vi "_OLS_Main_Rev3.vi"() -> ()   [LabVIEW 2024]
uses:
  Control Definitions/Def Results2.ctl
  Control Definitions/Def_ATPStatus.ctl
  Control Definitions/Def_PumpSpeed.ctl
  Control Definitions/Def TestState.ctl
  Control Definitions/DEF_CalConstants.ctl
  Control Definitions/Def PumpCtlRefs.ctl
  Control Definitions/Def CalTable.ctl
  Control Definitions/Def CalCoef.ctl
  Control Definitions/Registry Keys.ctl
  Control Definitions/Global 2.vi
  Control Definitions/Global 1.vi
panel:
  out "Cal Coef":T1
  in  "Cal Table":T2={"Level"={"LSf"=0.0, "LMf"=0.0, "LKf"=0.0, "LMe"=0.0, "LKe"=0.0, "LSe"=0.0}, "DataQ CH"=[{"RqLA"=0.5698, "RmLA"=102.56, "RqHA"=5.58, "RmHA"=981.0}, {"RqLA"=0.5707, "RmLA"=102.56, "RqHA"=5.5902, "RmHA"=978.2}]}
  out "ItemPath":string
  out "Laser (raw) 2":dbl=2.1254169074046554
  in  "End Prog":bool
  out "Test Index Out":i32=4
  out "PumpCtlRef out":T3
  out "Reg Cal Constants":T4={"Measure High"="0.000", "Laser High"="5.419", "Measure Low"="0.000", "Laser Low"="5.419", "Cal Name"="Rick", "Cal Date"="8/13/2024 3:15:10 PM", "Empty Inches"=8.0, "Full Inches"=2.6, "Valid"=FALSE}
  in  "Skip Pre-Lube":bool=TRUE
  out "TEST State Out":T5=enum."Wait1"
  in  "Pump Speed":T6=enum."STOP"
  in  "Num Chan":i32=2
  in  "VISA Refnum in":refnum<visa-resource-name>="COM3"
  in  "SimPV":bool
  out "Ch B  Sim":dbl=101.0
  out "Ch A  Sim":dbl=200.0
  out "Root Path":path=path "M:/OLS Level Test Project/PWC-OLS-Rev2/PWC-OLS"
  out "Time(ms)":dbl=7.099999999999983
  out "Level":bool=TRUE
  out "DataQ":bool
  in  "ChA":dbl(slide)=24.489795918367346 scale=0.0..1200.0
  in  "ChB":dbl(slide)=36.73469387755102 scale=0.0..1200.0
  in  "ChB +100":bool
  in  "ChA +100":bool
  in  "Check":bool
  out "Laser (raw)":dbl=2.1254169074046554
  out "Results out":T7=[[{"Fill"=0.0, "Drain"=0.0, "Status"=0, "Resistor"=100.0}, {"Fill"=8.52, "Drain"=0.0, "Status"=0, "Resistor"=101.0}], [{"Fill"=7.50499999999993, "Drain"=0.0, "Status"=4, "Resistor"=200.0}, {"Fill"=7.27499999999994, "Drain"=0.0, "Status"=0, "Resistor"=0.0}], [{"Fill"=0.0, "Drain"=0.0, "Status"=0, "Resistor"=0.0}, {"Fill"=0.0, "Drain"=0.0, "Status"=0, "Resistor"=0.0}], [{"Fill"=0.0, "Drain"=0.0, "Status"=0, "Resistor"=0.0}, {"Fill"=0.0, "Drain"=0.0, "Status"=0, "Resistor"=0.0}], [{"Fill"=0.0, "Drain"=0.0, "Status"=0, "Resistor"=0.0}, {"Fill"=0.0, "Drain"=0.0, "Status"=0, "Resistor"=0.0}], [{"Fill"=0.0, "Drain"=0.0, "Status"=0, "Resistor"=0.0}, {"Fill"=0.0, "Drain"=0.0, "Status"=0, "Resistor"=0.0}], [{"Fill"=0.0, "Drain"=0.0, "Status"=0, "Resistor"=0.0}, {"Fill"=0.0, "Drain"=0.0, "Status"=0, "Resistor"=0.0}], [{"Fill"=0.0, "Drain"=0.0, "Status"=0, "Resistor"=0.0}, {"Fill"=0.0, "Drain"=0.0, "Status"=0, "Resistor"=0.0}], [{"Fill"=0.0, "Drain"=0.0, "Status"=0, "Resistor"=0.0}, {"Fill"=0.0, "Drain"=0.0, "Status"=0, "Resistor"=0.0}], [{"Fill"=0.0, "Drain"=0.0, "Status"=0, "Resistor"=0.0}, {"Fill"=0.0, "Drain"=0.0, "Status"=0, "Resistor"=0.0}], [{"Fill"=0.0, "Drain"=0.0, "Status"=0, "Resistor"=0.0}, {"Fill"=0.0, "Drain"=0.0, "Status"=0, "Resistor"=0.0}]] {"Resistor" format="%.1f"; "Drain" format="%.3f"; "Fill" format="%.3f"}
  in  "DUT":i16=1
  in  "Pump JOG":bool
  in  "Run Test":bool=TRUE
  in  "Normal":cluster{u32, u32}[](array[cluster])=[{16711680, 1244948}]
  in  "Sim Color":cluster{u32, u32}[](array[cluster])=[{16774656, 1244948}]
  out "Level \nStatus":bool=TRUE
  out "DataQ\nStatus":bool
  in  "Level SP":dbl(slide)=7.46 scale=8.5..2.0
  in  "Level PV":dbl(slide)=7.459999999999936 scale=8.5..2.0
  out "Level":dbl=7.459999999999936 format="%.3f"
  in  "Drain":bool
  in  "Fill":bool
  in  "Simulate":bool=TRUE
  out "TEST NME":string="OLR001--"
  out "DataQ Input":T9(graph)={"ChA Ohms"=200.0, "ChB Ohms"=101.0, "Laser (raw)"=2.1254169074046554}
  out "Time Stamp":timestamp=timestamp(3807627813.1312256 s since 1904-01-01)
  in  "stop":bool
  out "ChB Ohms":dbl=101.0 format="%.1f"
  out "ChA Ohms":dbl=200.0 format="%.1f"
  # "Calibration & Scaling Table\n               Tank         Key          Ref\n               Scale        Level        Measure\nEmpty\n\n\nFull"
  # "8.5      1.7752      7.844\n\n2.0      6.112        3.511"
  # "CHA"
  # "CHB"
  # "ATP       Resistance     Fill        Drain"
  # "ATP       Resistance     Fill        Drain"
  # "Simulated Instrument Inputs"
  # "PUMP"
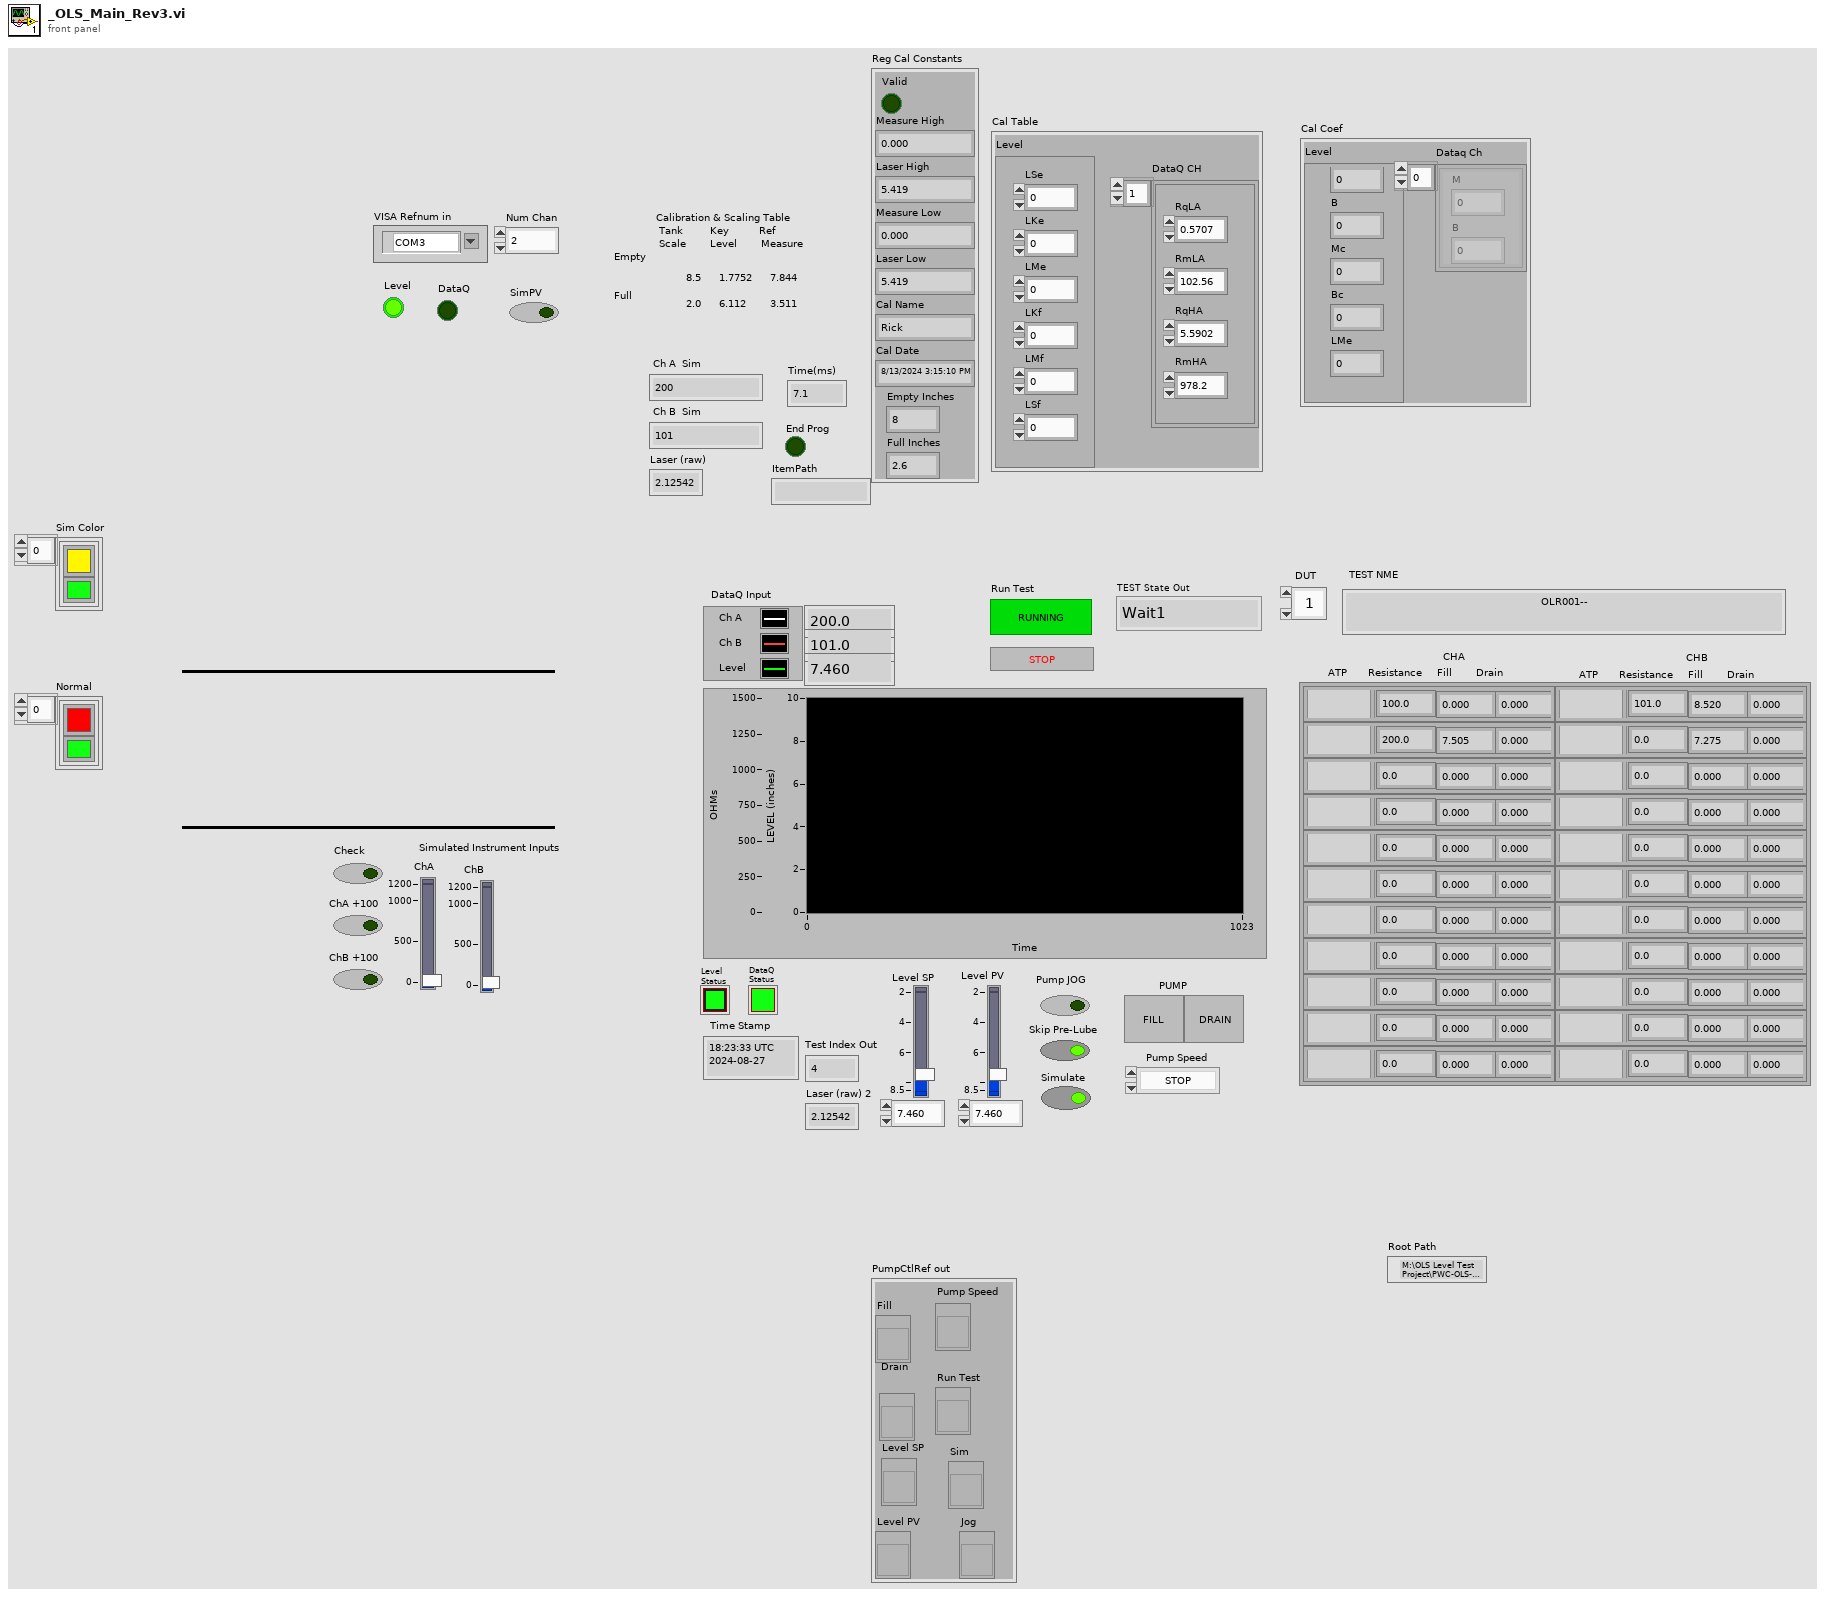
[diagram p1: front panel]
types:
  T1 = typedef "Def CalCoef.ctl" = cluster{"Level":cluster{"LMe":dbl, "Bc":dbl, "Mc":dbl, "B":dbl, "M":dbl}, "Dataq Ch":cluster{"B":dbl, "M":dbl}[]}
  T2 = typedef "Def CalTable.ctl" = cluster{"Level":cluster{"LSf":dbl, "LMf":dbl, "LKf":dbl, "LMe":dbl, "LKe":dbl, "LSe":dbl}, "DataQ CH":cluster{"RqLA":dbl, "RmLA":dbl, "RqHA":dbl, "RmHA":dbl}[]}
  T3 = typedef "Def PumpCtlRefs.ctl" = cluster{"Fill ":refnum<vi>, "Drain":refnum<vi>, "Level PV":refnum<vi>, "Pump Speed":refnum<vi>, "Run Test":refnum<vi>, "Sim":refnum<vi>, "Jog":refnum<vi>, "Level SP":refnum<vi>}
  T4 = typedef "DEF_CalConstants.ctl" = cluster{"Measure High":string, "Laser High":string, "Measure Low":string, "Laser Low":string, "Cal Name":string, "Cal Date":string, "Empty Inches":dbl, "Full Inches":dbl, "Valid":bool}
  T5 = typedef "Def TestState.ctl" = enum16{"MANUAL", "Start", "Pre-Fill", "Pre-Fill Measure", "Pre-Drain", "Pre-Drin Measure", "Init-Record", "Load Fill Spec", "Filling Hi", "Wait1", "Record Fill", "Load Drain Spec", "Draining Lo", "Wait2", "Record Drain", "Empty", "Done"}
  T6 = typedef "Def_PumpSpeed.ctl" = enum16{"FAST", "SLOW", "CREEP", "STOP"}
  T7 = typedef "Def Results2.ctl" = cluster{"Fill":dbl, "Drain":dbl, "Status":T8, "Resistor":dbl}[][]
  T8 = typedef "Def_ATPStatus.ctl" = i16
  T9 = cluster{"ChA Ohms":dbl, "ChB Ohms":dbl, "Laser (raw)":dbl}
  T10 = typedef "Registry Keys.ctl" = enum16{"Report Files Key", "Config Files Key"}
  T11 = cluster{"Level \nStatus":refnum<vi>, "DataQ\nStatus":refnum<vi>}
  T12 = typedef "Def FullCfg.ctl" = cluster{"Bench Config":T13, "Test Value Table ":dbl[][], "Table Col Titles":string[][], "cluster":T3, "Bench Status":T14}
  T13 = typedef "Def BenchCfg.ctl" = cluster{"Name":string, cluster{"Step Levels":dbl, "Tolerance":dbl, "Sample Rate":dbl, "Resistor":dbl, "M Level Cal":dbl, "[B Level Cal":dbl, "Max Fill Rate":dbl, "Empty Inches":dbl, "Full Inches":dbl}}
  T14 = typedef "Def Bench Status.ctl" = cluster{"Pump Status":refnum<vi>, "Instrumnet\n Status":refnum<vi>}
  T15 = enum16{"MANUAL", "Start", "Filling", "FULL", "Draining", "EMPTY", "Done"}
  T16 = cluster{"Resistor":dbl, "Fill":dbl, "Drain":dbl, "Status":i16}
  T17 = cluster{"Resistor":dbl, "Fill":dbl, "Drain":dbl, "Status":i16}[][]
  T18 = typedef "DEF_SpecsOut.ctl" = cluster{"aSpecsTable":T19[], "Pump CtlRef In":T3, "TEST State Out":T5, "TEST Index":i32, "Drain!Fill":bool}
  T19 = typedef "Def Spec RNG.ctl" = cluster{"Specs":dbl[], "LUT Status":T20}
  T20 = typedef "Ded LUT_Status.ctl" = cluster{"ChA/!ChB":bool, "Drain/!Fill":bool, "In Range?":bool, "Switch Range?":bool, "Measure R?":bool, "Vaild R?":bool, "Index(n)":i32, "Index(n)-1":i32, "Index Max":i32, "Index(n-1)":i32}
  T21 = typedef "Def Measure.ctl" = cluster{"ChA R":dbl, "ChB R":dbl, "Level PV":dbl}
  T22 = cluster{"Resistor":dbl, "Fill":dbl, "Drain":dbl, "Resistor":dbl}[][]
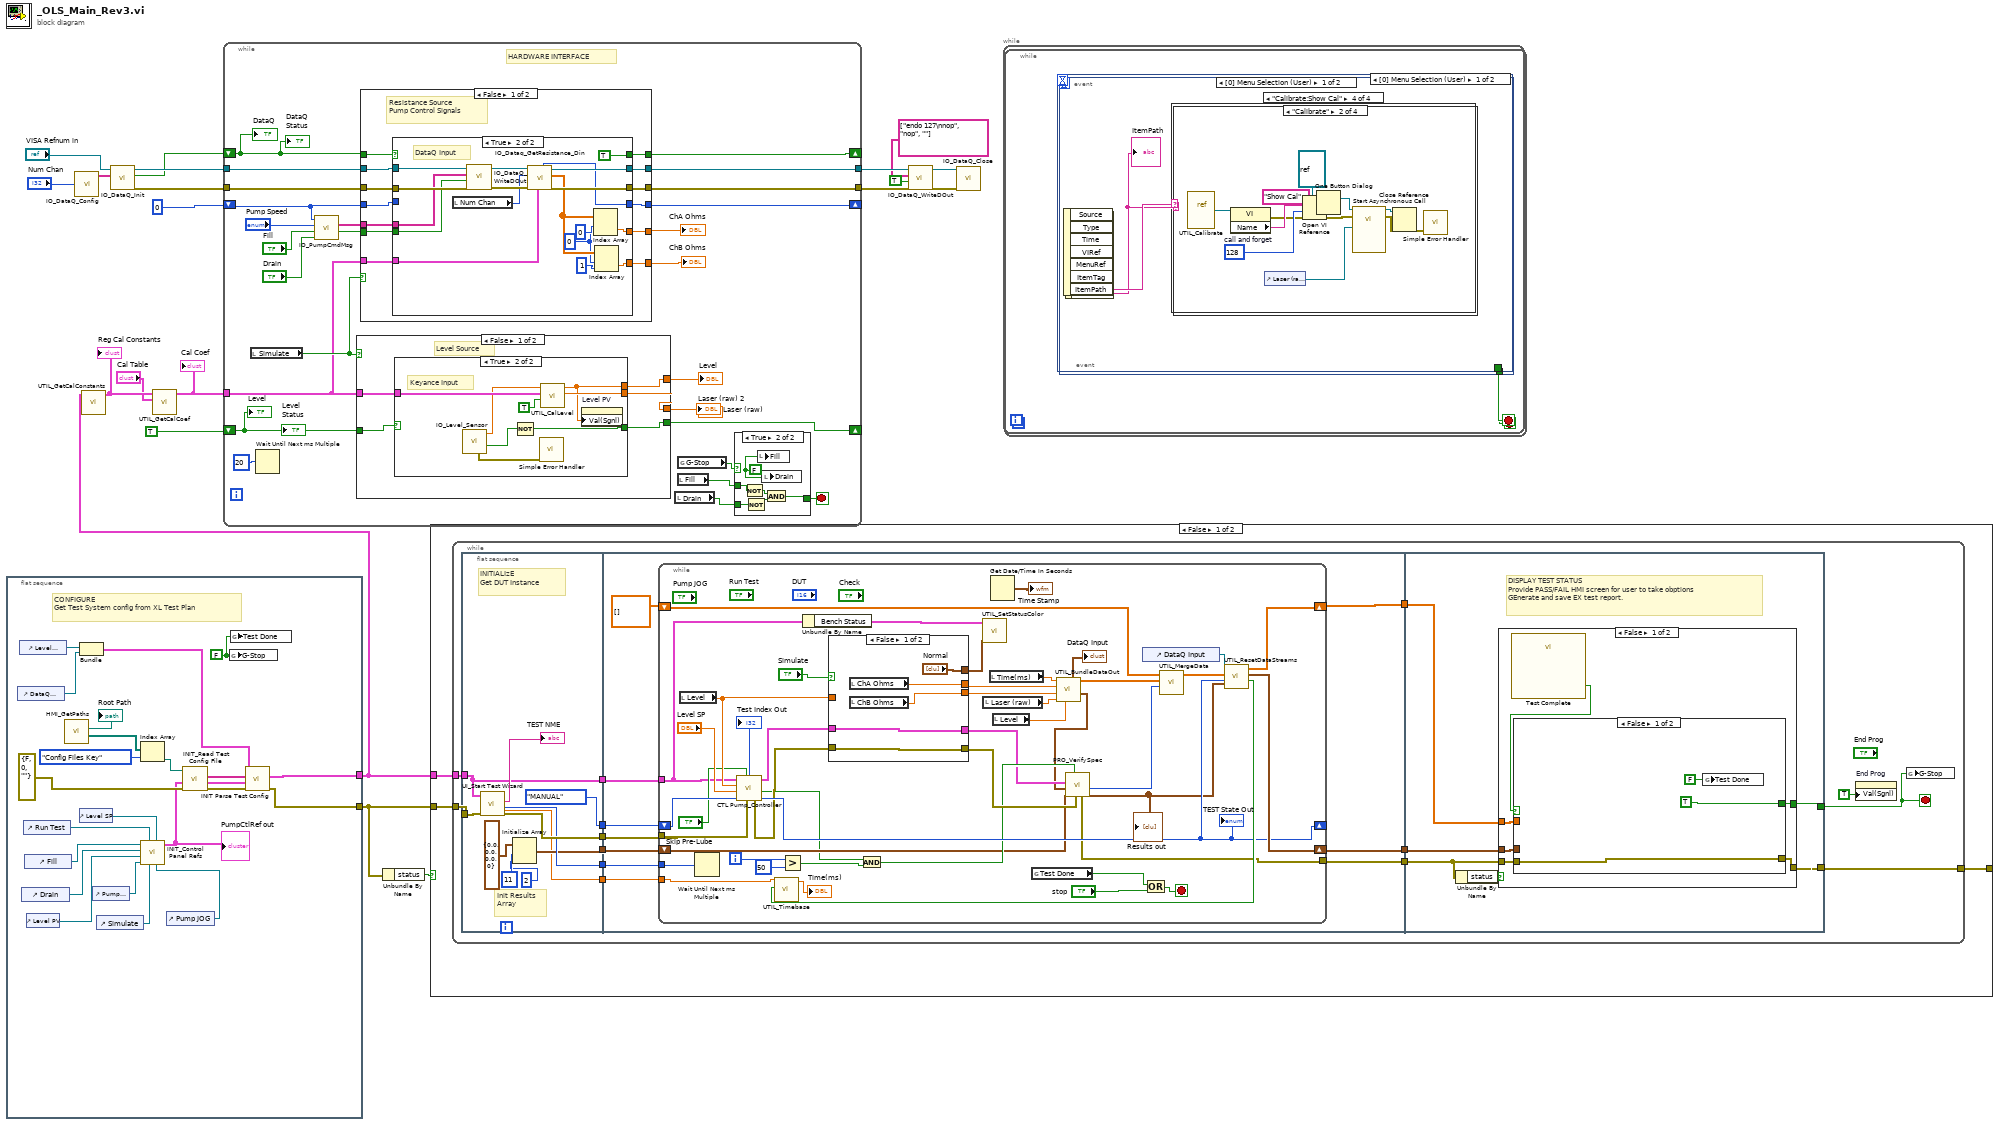
[diagram p0: block diagram]
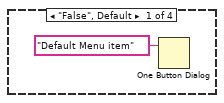
[diagram p2: hidden frame]
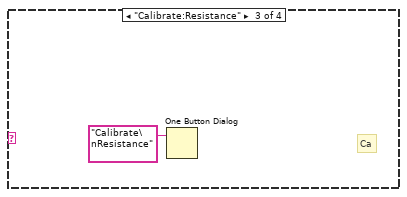
[diagram p3: hidden frame]
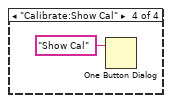
[diagram p4: hidden frame]
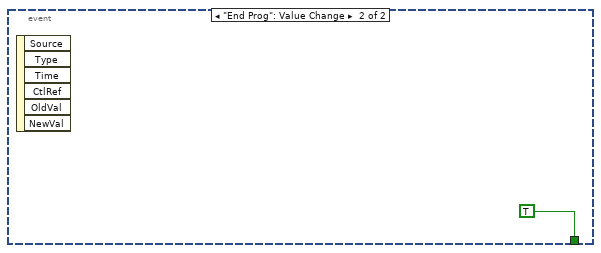
[diagram p5: hidden frame]
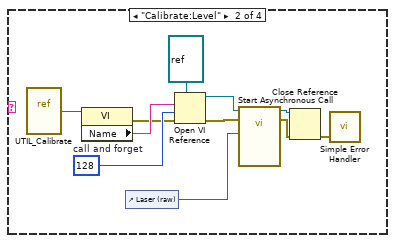
[diagram p7: hidden frame]
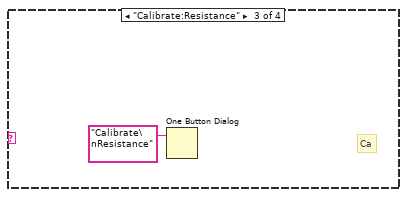
[diagram p8: hidden frame]
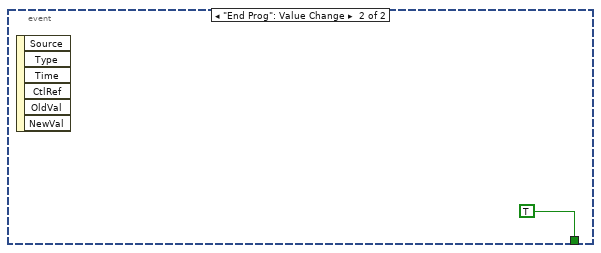
[diagram p9: hidden frame]
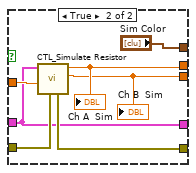
[diagram p10: hidden frame]
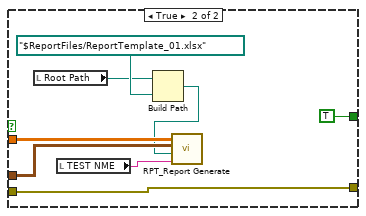
[diagram p11: hidden frame]
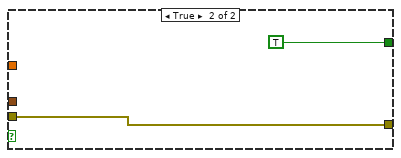
[diagram p12: hidden frame]
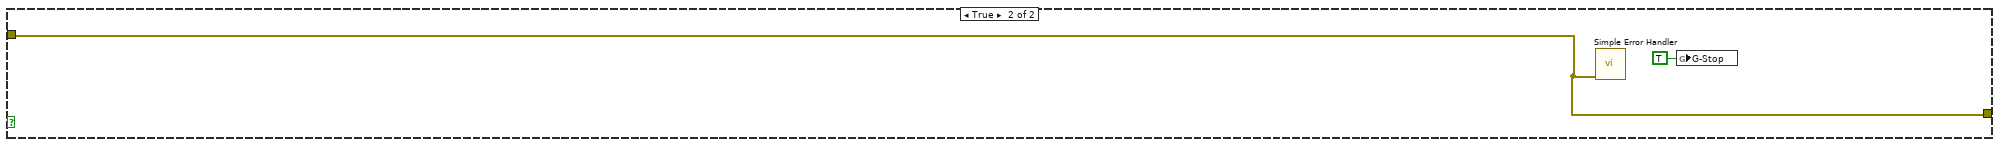
[diagram p13: hidden frame]
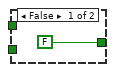
[diagram p14: hidden frame]
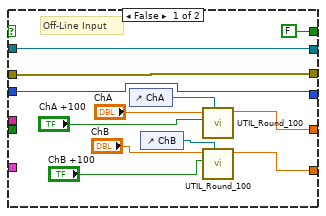
[diagram p15: hidden frame]
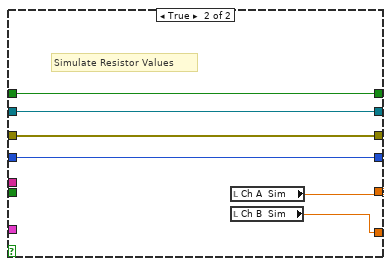
[diagram p16: hidden frame]
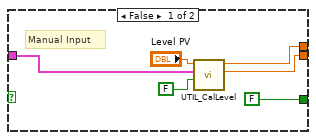
[diagram p17: hidden frame]
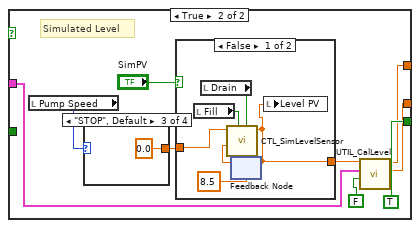
[diagram p18: hidden frame]
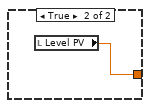
[diagram p19: hidden frame]
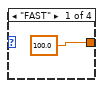
[diagram p20: hidden frame]
diagram:
  n1 = flat-sequence {
    tunnel: [w40] -> w14
    tunnel: [w32] -> w3
    frame #0 {
      w27 = FALSE ("G-Stop")
      # "CONFIGURE\nGet Test System config from XL Test Plan"
      n2 = control-ref of="DataQ\nStatus"() -> (w29:refnum<vi>)
      n3 = control-ref of="Level \nStatus"() -> (w39:refnum<vi>)
      n4 = control-ref of="Drain"() -> (w41:refnum<vi>)
      n5 = control-ref of="Run Test"() -> (w34:refnum<vi>)
      n6 = control-ref of="Fill"() -> (w35:refnum<vi>)
      n7 = control-ref of="Level PV"() -> (w37:refnum<vi>)
      n8 = call "HMI_GetPaths.vi"() -> ("Default Paths"=w22:path[], "Root Path"=→"Root Path":path)  [unwired: 10 in]
      n9 = Bundle("Level \nStatus"=w39, "DataQ\nStatus"=w29) -> (w38:T11)  [unwired: 1 in]
      n10 = control-ref of="Level SP"() -> (w28:refnum<vi>)
      n11 = control-ref of="Pump Speed"() -> (w24:refnum<vi>)
      n12 = control-ref of="Simulate"() -> (w31:refnum<vi>)
      n13 = Index Array(array=w22, index=Registry_Keys."Config Files Key" ("Reg Key")) -> (element=w21:path)
      n14 = control-ref of="Pump JOG"() -> (w30:refnum<vi>)
      n15 = call "INIT_Control Panel Refs.vi"("Jog"=w30, "Level SP"=w28, "Sim"=w31, "Run Test"=w34, "Pump Speed"=w24, "Level PV"=w37, "Drain"=w41, "Fill"=w35) -> ("PumpCtlRef out"=w25:T3)  [unwired: 3 in]
      "PumpCtlRef out" <- w25
      n16 = call "INIT_Read Test Config File.vi"("error in (no error)"=errorcluster {"status"=FALSE, "code"=0, "source"=""}, "Path"=w21) -> ("error out 2"=w33:errorcluster, "Config\nFile Data"=w36:string[][])  [unwired: 8 in]
      n17 = global write "Global 1.vi" "G-Stop"(w27) -> ()
      n18 = global write "Global 2.vi" "Test Done"(w27) -> ()
      n19 = call "INIT Parse Test Config.vi"("error in (no error)"=w33, "Pump CtlRef In"=w25, "All XL Input"=w36, "Bench Status"=w38) -> ("error out"=w40:errorcluster, "Full Config"=w32:T12)  [unwired: 5 in, 1 out]
    }
  }
  n20 = call "IO_DataQ_Config.vi"("Num Chan"="Num Chan") -> ("Init Message"=w20:string[])  [unwired: 10 in]
  n21 = call "UTIL_GetCalConstants.vi"("Full Config"=w3) -> ("Cal Constants"=w4:T4)  [unwired: 9 in, 1 out]
  "Reg Cal Constants" <- w4
  n22 = call "IO_DataQ_Init.vi"("Command\nList"=w20, "VISA Refnum in"="VISA Refnum in") -> ("error out"=w18:errorcluster, "Connected?"=w17:bool, "VISA resource name out"=w19:refnum<visa-resource-name>)  [unwired: 7 in]
  n23 = call "UTIL_GetCalCoef.vi"("Cal Table"="Cal Table", "Cal Constants"=w4) -> ("Cal Coef"=w1:T1)  [unwired: 9 in]
  "Cal Coef" <- w1
  n24 = while {
    shift-right: [w65] -> _
    shift-left: TRUE ("Pump \nStatus") -> [w47]
    tunnel: w19 -> [w64]
    tunnel: w18 -> [w63]
    tunnel: [w61] -> w13
    tunnel: [w62] -> w11
    shift-right: [w60] -> _
    shift-left: w17 -> [w59]
    tunnel: w1 -> [w43]
    shift-right: [w50] -> _
    shift-left: 0 -> [w46]
    stop <- w55 stop-if-true
    # "HARDWARE INTERFACE"
    n25 = local read "Simulate"() -> (w57:bool)
    n26 = Wait Until Next ms Multiple(millisecond multiple=u32 20) -> ()  [unwired: 1 out]
    n27 = call "IO_PumpCmdMsg.vi"("Drain Signal"="Drain", "FIll Signal"="Fill", "Pump Speed"="Pump Speed", "Cmd IN"=w46) -> ("Msg Active"=w44:bool, "Message"=w58:string[])  [unwired: 4 in, 2 out]
    n28 = case shown="False" w57 {
      tunnel: [w129 w149] -> w45
      tunnel: [w128 w151] -> w66
      tunnel: [w125 TRUE] -> w65
      tunnel: w47 -> [w127 _]
      tunnel: w43 -> [w126 w144]
      frame False {
        # "Level Source"
        n29 = case shown="True" w127 {
          tunnel: [w133 w136] -> w129
          tunnel: [w132 w141] -> w128
          tunnel: [FALSE ("status") w140] -> w125
          tunnel: w126 -> [w134 w142]
          frame False {
            # "Manual Input"
            n30 = call "UTIL_CalLevel.vi"("Key is In?"=FALSE, "Cal Coef"=w134, "Input"="Level PV") -> ("PVc"=w132:dbl, "PVs"=w133:dbl)  [unwired: 7 in]
          }
          frame True {
            # "Keyance Input"
            n31 = call "IO_Level_Sensor.vi"() -> ("status"=w138:bool, "PV (raw)"=w139:dbl, "error OUT"=w137:errorcluster)  [unwired: 9 in]
            n32 = Not(x=w138) -> (.not. x?=w140:bool)
            n33 = call <vilib>:"Simple Error Handler.vi"("error in (no error)"=w137) -> ()  [unwired: 4 in, 5 out]
            n34 = call "UTIL_CalLevel.vi"("Key is In?"=TRUE, "Cal Coef"=w142, "Input"=w139) -> ("PVc"=w141:dbl, "PVs"=w136:dbl)  [unwired: 7 in]
            n35 = property on="Level PV" class="Slide (strict)"("Val(Sgnl)"=w136) -> ()  [unwired: 2 in, 2 out]
          }
        }
      }
      frame True {
        # "Simulated Level"
        n36 = local read "Pump Speed"() -> (w147:T6)
        n37 = case shown="\"STOP\", Default" w147 {
          tunnel: [100.0 ("Ctl Sig") 5.0 ("Ctl Sig") 0.0 ("Ctl Sig") 50.0 ("Ctl Sig")] -> w148
          frame "FAST" {
          }
          frame "CREEP" {
          }
          frame "STOP", Default {
          }
          frame "SLOW" {
          }
        }
        n38 = case shown="False" "SimPV" {
          tunnel: w148 -> [w157 _]
          tunnel: [w153 w159] -> w146
          frame False {
            n39 = local read "Fill"() -> (w158:bool)
            n40 = local read "Drain"() -> (w154:bool)
            n41 = feedback #1(8.5 ("PV Level Inch")) -> (w155:dbl)
            n42 = call "CTL_SimLevelSensor.vi"("Drain IN"=w154, "Fill IN"=w158, "Level PV in"=w155, "Pump Speed"=w157) -> ("PV Level Inch"=w153:dbl)  [unwired: 7 in]
            n43 = feedback-in #1(w153) -> ()
            n44 = local write "Level PV"(w153) -> ()
          }
          frame True {
            n45 = local read "Level PV"() -> (w159:dbl)
          }
        }
        n46 = call "UTIL_CalLevel.vi"("Key is In?"=FALSE, "Cal Coef"=w144, "Input"=w146) -> ("PVc"=w151:dbl, "PVs"=w149:dbl)  [unwired: 7 in]
      }
    }
    "Level" <- w45
    "Laser (raw)" <- w66
    n47 = case shown="False" w57 {
      tunnel: [w88 w121] -> w67
      tunnel: [w87 w120] -> w48
      tunnel: w64 -> [w80 w123]
      tunnel: w63 -> [w82 w122]
      tunnel: [w86 w122] -> w62
      tunnel: [w85 w123] -> w61
      tunnel: [w84 w124] -> w60
      tunnel: w59 -> [w83 w124]
      tunnel: w58 -> [w81 _]
      tunnel: w44 -> [w79 _]
      tunnel: [w78 w119] -> w50
      tunnel: w46 -> [w77 w119]
      tunnel: w43 -> [w76 _]
      frame False {
        # "Resistance Source\nPump Control Signals"
        n48 = case shown="True" w83 {
          tunnel: [w93 w115] -> w88
          tunnel: [w94 w104] -> w87
          tunnel: [w95 w118] -> w85
          tunnel: [w96 w117] -> w86
          tunnel: [FALSE TRUE] -> w84
          tunnel: w82 -> [w96 w113]
          tunnel: w81 -> [_ w109]
          tunnel: w80 -> [w95 w112]
          tunnel: w79 -> [_ w108]
          tunnel: [w89 w105] -> w78
          tunnel: w77 -> [w89 _]
          tunnel: w76 -> [_ w101]
          frame False {
            # "Off-Line Input"
            n49 = control-ref of="ChA"() -> (w92:refnum<vi>)
            n50 = control-ref of="ChB"() -> (w90:refnum<vi>)
            n51 = call "UTIL_Round_100.vi"("Num Refnum"=w92, "100"="ChA +100", "IN"="ChA") -> ("OUT"=w94:dbl)  [unwired: 8 in]
            n52 = call "UTIL_Round_100.vi"("Num Refnum"=w90, "100"="ChB +100", "IN"="ChB") -> ("OUT"=w93:dbl)  [unwired: 8 in]
          }
          frame True {
            w103 = 0 ("disabled index (col)")
            # "DataQ Input"
            n53 = local read "Num Chan"() -> (w106:i32)
            n54 = call "IO_DataQ_WriteDOut.vi"("error in (no error)"=w113, "Msg Active"=w108, "Message"=w109, "VISA Refnum in"=w112) -> ("error out"=w111:errorcluster, "VISA Refnum out"=w110:refnum<visa-resource-name>)  [unwired: 6 in]
            n55 = call "IO_Dataq_GetResistance_Din.vi"("Cal Coef"=w101, "error in (no error)"=w111, "Num Chan"=w106, "VISA Refnum in"=w110) -> ("error out"=w117:errorcluster, "Analog"=w107:dbl[][], "VISA Refnum out"=w118:refnum<visa-resource-name>, "Cmd"=w105:u32)  [unwired: 2 in, 2 out]
            n56 = Index Array(array=w107, index (row)=0 ("index"), index (col)=w103) -> (element=w104:dbl)
            n57 = Index Array(array=w107, index (row)=w103, index (col)=1 ("index")) -> (element=w115:dbl)
          }
        }
      }
      frame True {
        # "Simulate Resistor Values"
        n58 = local read "Ch A  Sim"() -> (w120:dbl)
        n59 = local read "Ch B  Sim"() -> (w121:dbl)
      }
    }
    "ChA Ohms" <- w48
    "ChB Ohms" <- w67
    n60 = local read "Drain"() -> (w53:bool)
    n61 = local read "Fill"() -> (w54:bool)
    n62 = global read "Global 1.vi" "G-Stop"() -> (w56:bool)
    n63 = case shown="True" w56 {
      tunnel: [FALSE w71] -> w55
      tunnel: w54 -> [_ w73]
      tunnel: w53 -> [_ w70]
      frame False {
      }
      frame True {
        w75 = FALSE
        n64 = Not(x=w73) -> (.not. x?=w74:bool)
        n65 = Not(x=w70) -> (.not. x?=w72:bool)
        n66 = local write "Fill"(w75) -> ()
        n67 = local write "Drain"(w75) -> ()
        n68 = And(x=w74, y=w72) -> (x .and. y?=w71:bool)
      }
    }
    "DataQ\nStatus" <- w59
    "Level \nStatus" <- w47
    "DataQ" <- w59
    "Level" <- w47
  }
  n69 = Unbundle By Name(w14) -> ("status"=w16:bool)
  n70 = case shown="False" w16 {
    tunnel: w14 -> [w166 w284]
    tunnel: w3 -> [w165 _]
    tunnel: [w164 w284] -> _
    frame False {
      n71 = while {
        tunnel: w166 -> [w177]
        tunnel: w165 -> [w175]
        tunnel: [w170] -> w164
        stop <- w168 stop-if-true
        n72 = flat-sequence {
          tunnel: [w189] -> w179
          tunnel: [w190] -> w178
          tunnel: w177 -> [w191]
          tunnel: [w181] -> w176
          tunnel: w175 -> [w181]
          tunnel: [T15."MANUAL" ("TEST STATUS Out")] -> w174
          tunnel: [w184] -> w173
          tunnel: [w183] -> w169
          tunnel: [w195] -> w180
          tunnel: w179 -> [w200]
          tunnel: w178 -> [w201]
          tunnel: w176 -> [w192]
          tunnel: w174 -> [w193]
          tunnel: w173 -> [w199]
          tunnel: [w198] -> w172
          tunnel: [w197] -> w171
          tunnel: w169 -> [w196]
          tunnel: w180 -> [w264]
          tunnel: [w263] -> w168
          tunnel: [w261] -> w170
          tunnel: w172 -> [w260]
          tunnel: w171 -> [w259]
          frame #0 {
            # "Init Results\nArray"
            # "INITIALIzE\nGet DUT Instance"
            n73 = call "UI_Start Test Wizard.vi"("error in (no error)"=w191, "Full Config"=w181) -> ("error out"=w190:errorcluster, "Time Base mS"=w189:i32, "Title"=→"TEST NME":string, "Sample Rate"=w183:dbl)  [unwired: 4 in]
            n74 = Initialize Array(T16 {"Resistor"=0.0, "Fill"=0.0, "Drain"=0.0, "Status"=0} ("Cluster 2"), 11 ("dimension size"), 2 ("dimension size")) -> (w184:T17)
          }
          frame #1 {
            n75 = while {
              tunnel: w200 -> [w244]
              tunnel: w201 -> [w233]
              tunnel: [w220] -> w195
              shift-right: [w227] -> w197
              shift-left: w199 -> [w219]
              tunnel: w196 -> [w232]
              shift-right: [w228] -> w198
              shift-left: dbl[][] [] ("Array") -> [w213]
              shift-right: [w224] -> _
              shift-left: w193 -> [w223]
              tunnel: w192 -> [w203]
              i -> [w231]
              stop <- w241 stop-if-true
              n76 = local read "Level"() -> (w208:dbl)
              n77 = Wait Until Next ms Multiple(millisecond multiple=w244) -> ()  [unwired: 1 out]
              n78 = call "CTL Pump_Controller.vi"("error in (no error)"=w233, "Skip Pre-Lub"="Skip Pre-Lube", "TEST State In"=w223, "Level SP"="Level SP", "Level PV"=w208, "Full Cfg 2"=w203) -> ("TEST State Out"=w224:T5, "Enable"=w204:bool, "Specs Out"=w206:T18, "error out"=w205:errorcluster, "Test Index Out"=→"Test Index Out":i32)  [unwired: 1 in]
              "TEST State Out" <- w224
              n79 = Greater?(x=w231, y=50) -> (0:w229:bool)
              n80 = Unbundle By Name(w203) -> ("Bench Status"=w242:T14)
              n81 = case shown="False" "Simulate" {
                tunnel: w205 -> [w251 w254]
                tunnel: [w251 w257] -> w222
                tunnel: ["Normal" "Sim Color"] -> w243
                tunnel: [w249 w256] -> w236
                tunnel: [w248 w255] -> w235
                tunnel: w206 -> [w247 w252]
                tunnel: w208 -> [_ w253]
                tunnel: [w247 w252] -> w218
                frame False {
                  n82 = local read "ChA Ohms"() -> (w249:dbl)
                  n83 = local read "ChB Ohms"() -> (w248:dbl)
                }
                frame True {
                  n84 = call "CTL_Simulate Resistor.vi"("error in (no error)"=w254, "Level IN"=w253, "Specs IN"=w252) -> ("Ch B  Ohms"=w255:dbl, "Ch A  Ohms"=w256:dbl, "error out"=w257:errorcluster)  [unwired: 6 in]
                  "Ch A  Sim" <- w256
                  "Ch B  Sim" <- w255
                }
              }
              n85 = And(x=w204, y=w229) -> (x .and. y?=w221:bool)
              n86 = call "UTIL_SetStatusColor.vi"("Colors [4] in"=w243, "Bench Status"=w242) -> ()  [unwired: 10 in]
              n87 = local read "Laser (raw)"() -> (w237:dbl)
              n88 = local read "Time(ms)"() -> (w238:dbl)
              n89 = Get Date/Time In Seconds() -> (seconds since 1Jan1904=→"Time Stamp":timestamp)
              n90 = local read "Level"() -> (w209:dbl)
              n91 = global read "Global 2.vi" "Test Done"() -> (w239:bool)
              n92 = call "UTIL_BundleDataOut.vi"("Level PV"=w209, "Laser (raw)"=w237, "ChB Ohms"=w235, "ChA Ohms"=w236, "Time (ms)"=w238) -> ("Measure"=w217:T21, "Data Out"=w215:dbl[], "Chart Data"=→"DataQ Input":T9)  [unwired: 3 in, 1 out]
              n93 = call "PRO_VerifySpec.vi"("error in (no error)"=w222, "Enable"=w221, "Results in"=w219, "Measure In"=w217, "Specs In"=w218) -> ("Results out"=w216:T7, "Status Code"=w214:i32, "error out"=w220:errorcluster)  [unwired: 4 in]
              "Results out" <- w216
              n94 = control-ref of="DataQ Input"() -> (w210:refnum<vi>)
              n95 = Or(x=w239, y="stop") -> (x .or. y?=w241:bool)
              n96 = call "UTIL_MergeData.vi"("Status Code"=w214, "New Data"=w215, "Data In"=w213) -> ("Data out"=w212:dbl[][])  [unwired: 8 in]
              n97 = call "UTIL_ResetDataStreams.vi"("Results in"=w216, "TEST State Out"=w224, "Data in"=w212, "WaveformChart in"=w210) -> ("Value (Signaling)"=w225:bool, "Results out 2"=w227:T22, "Array"=w228:dbl[][])  [unwired: 5 in]
              n98 = call "UTIL_Timebase.vi"("Reset"=w225, "Sample Rate"=w232) -> ("Time(ms)"=→"Time(ms)":dbl)  [unwired: 9 in]
            }
          }
          frame #2 {
            # "DISPLAY TEST STATUS\nProvide PASS/FAIL HMI screen for user to take obptions\nGEnerate and save EX test report."
            n99 = Unbundle By Name(w264) -> ("status"=w262:bool)
            n100 = case shown="False" w262 {
              tunnel: w264 -> [w268 w282]
              tunnel: [w269 TRUE] -> w263
              tunnel: [w267 w282] -> w261
              tunnel: w260 -> [w266 _]
              tunnel: w259 -> [w265 _]
              frame False {
                n101 = call "Test Complete"() -> ("SAVE"=w270:bool)  [unwired: 18 in, 1 out]
                n102 = case shown="False" w270 {
                  tunnel: [TRUE TRUE] -> w269
                  tunnel: w268 -> [w272 w280]
                  tunnel: [w272 w280] -> w267
                  tunnel: w266 -> [_ w279]
                  tunnel: w265 -> [_ w278]
                  frame False {
                    n103 = global write "Global 2.vi" "Test Done"(FALSE ("Test Done")) -> ()
                  }
                  frame True {
                    n104 = local read "Root Path"() -> (w276:path)
                    n105 = local read "TEST NME"() -> (w274:string)
                    n106 = Build Path(base path=w276, name or relative path=path "$ReportFiles/ReportTemplate_01.xlsx") -> (appended path=w275:path)
                    n107 = call "RPT_Report Generate.vi"("Report Name"=w274, "template"=w275, "Results"=w278, "Wave Data"=w279) -> ()  [unwired: 8 in]
                  }
                }
              }
              frame True {
              }
            }
          }
        }
        n108 = property on="End Prog" class="Bool (strict)"("Val(Sgnl)"=TRUE ("End Prog")) -> ()  [unwired: 2 in, 2 out]
        n109 = global write "Global 1.vi" "G-Stop"(w168) -> ()
      }
    }
    frame True {
      n110 = call <vilib>:"Simple Error Handler.vi"("error in (no error)"=w284) -> ()  [unwired: 4 in, 5 out]
      n111 = global write "Global 1.vi" "G-Stop"(TRUE ("G-Stop")) -> ()
    }
  }
  n112 = call "IO_DataQ_WriteDOut.vi"("error in (no error)"=w11, "Msg Active"=TRUE, "Message"=string[] ["endo 127\nnop", "nop", ""], "VISA Refnum in"=w13) -> ("error out"=w10:errorcluster, "VISA Refnum out"=w12:refnum<visa-resource-name>)  [unwired: 6 in]
  n113 = call "IO_DataQ_Close.vi"("error in"=w10, "VISA resource name"=w12) -> ()  [unwired: 10 in]
  n114 = while {
    stop <- w286 stop-if-true
    n115 = event shown="[0] Menu Selection (User)" {
      selector: _ -> [_ _]
      dyn-events: _ -> [_ _]
      timeout: _ -> [_ _]
      tunnel: [_ TRUE] -> w286
      event Menu Selection (User) {
        n116 = event-data() -> ("ItemPath"=w287:string)  [unwired: 1 in, 6 out]
        n117 = case shown="\"Calibrate:Show Cal\"" w287 {
          frame "False", Default {
          }
          frame "Calibrate:Level" {
            w298 = 128  # call and forget
            n118 = vi-ref "UTIL_Calibrate.vi"() -> (w291:refnum<vi>)
            n119 = property class="VI"(reference=w291) -> (error out=w289:errorcluster, "Name"=w290:string)  [unwired: 1 in, 1 out]
            n120 = control-ref of="Laser (raw)"() -> (w288:refnum<vi>)
            n121 = Open VI Reference(type specifier VI Refnum (for type only)=refnum<vi> refnum, vi path=w290, options=w298, error in (no error)=w289) -> (vi reference=w296:refnum<vi>, error out=w295:errorcluster)  [unwired: 2 in]
            n122 = call-by-ref "Start Asynchronous Call"(reference=w296, error in=w295, "Digital in"=w288) -> (reference out=w293:refnum<vi>, error out=w294:errorcluster)  [unwired: 10 in, 1 out]
            n123 = Close Reference(reference=w293, error in (no error)=w294) -> (error out=w292:errorcluster)
            n124 = call <vilib>:"Simple Error Handler.vi"("error in (no error)"=w292) -> ()  [unwired: 4 in, 5 out]
          }
          frame "Calibrate:Resistance" {
            # "Ca"
            n125 = One Button Dialog(message="Calibrate\nResistance") -> ()  [unwired: 1 in, 1 out]
          }
          frame "Calibrate:Show Cal" {
            n126 = One Button Dialog(message="Show Cal") -> ()  [unwired: 1 in, 1 out]
          }
        }
      }
      event "End Prog": Value Change {
        n127 = event-data() -> ()  [unwired: 1 in, 6 out]
      }
    }
  }
  n128 = while {
    stop <- w302 stop-if-true
    n129 = event shown="[0] Menu Selection (User)" {
      selector: _ -> [_ _]
      dyn-events: _ -> [_ _]
      timeout: _ -> [_ _]
      tunnel: [_ TRUE] -> w302
      event Menu Selection (User) {
        n130 = event-data() -> ("ItemPath"=w303:string)  [unwired: 1 in, 6 out]
        "ItemPath" <- w303
        n131 = case shown="\"Calibrate\"" w303 {
          frame "False", Default {
            n132 = One Button Dialog(message="Default Menu item") -> ()  [unwired: 1 in, 1 out]
          }
          frame "Calibrate" {
            w315 = 128  # call and forget
            n133 = vi-ref "UTIL_Calibrate.vi"() -> (w308:refnum<vi>)
            n134 = property class="VI"(reference=w308) -> (error out=w306:errorcluster, "Name"=w307:string)  [unwired: 1 in, 1 out]
            n135 = control-ref of="Laser (raw) 2"() -> (w305:refnum<vi>)
            n136 = Open VI Reference(type specifier VI Refnum (for type only)=refnum<vi> refnum, vi path=w307, options=w315, error in (no error)=w306) -> (vi reference=w313:refnum<vi>, error out=w312:errorcluster)  [unwired: 2 in]
            n137 = call-by-ref "Start Asynchronous Call"(reference=w313, error in=w312, "Digital in"=w305) -> (reference out=w310:refnum<vi>, error out=w311:errorcluster)  [unwired: 10 in, 1 out]
            n138 = Close Reference(reference=w310, error in (no error)=w311) -> (error out=w309:errorcluster)
            n139 = call <vilib>:"Simple Error Handler.vi"("error in (no error)"=w309) -> ()  [unwired: 4 in, 5 out]
          }
          frame "Calibrate:Resistance" {
            # "Ca"
            n140 = One Button Dialog(message="Calibrate\nResistance") -> ()  [unwired: 1 in, 1 out]
          }
          frame "Calibrate:Show Cal" {
            n141 = One Button Dialog(message="Show Cal") -> ()  [unwired: 1 in, 1 out]
          }
        }
      }
      event "End Prog": Value Change {
        n142 = event-data() -> ()  [unwired: 1 in, 6 out]
      }
    }
  }
